vi "TCP通讯.vi"(7 "service name":string caption="服务名称", 8 "error in":errorcluster caption="错误输入（无错误）", 9 "数据输入":string, 10 "选项":enum16{"NA", "侦听", "读取", "写入", "关闭", "打开TCP连接"}(ring)=enum."侦听", 11 "connection ID in":refnum<k5>) -> (0 "error out":errorcluster caption="错误输出", 1 "数据输出":string, 2 "send ok":bool, 3 "connection ID out":refnum<k5>, 4 "open com":bool)   [LabVIEW 2017]
panel:
  out "写入的字节":i32
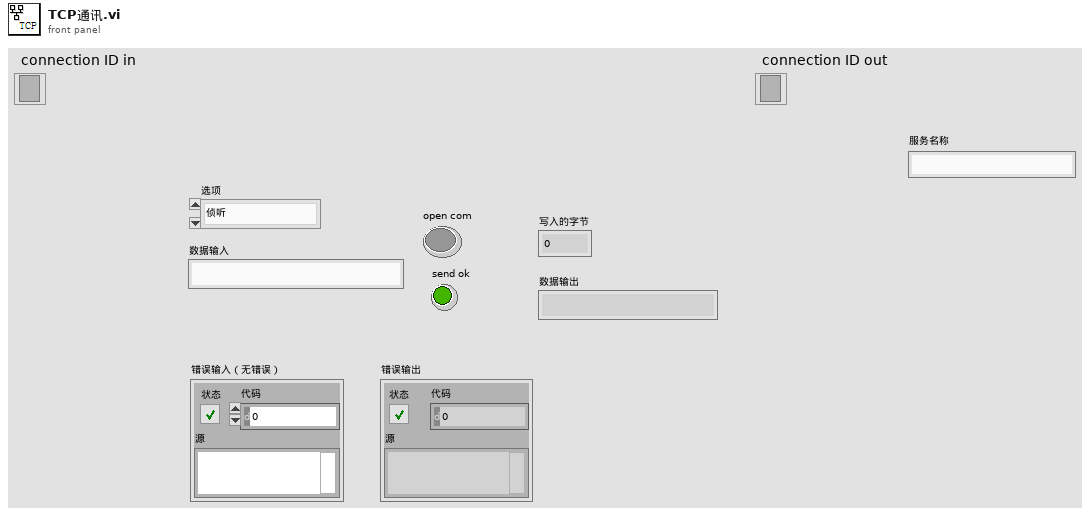
[diagram p1: front panel]
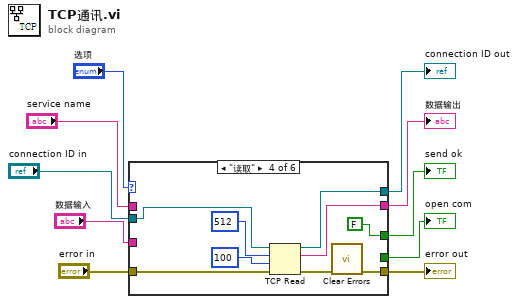
[diagram p0: block diagram]
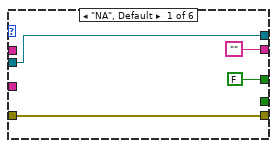
[diagram p2: hidden frame]
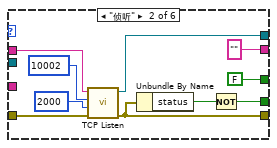
[diagram p3: hidden frame]
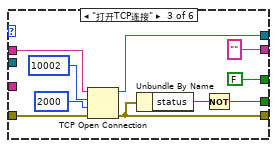
[diagram p4: hidden frame]
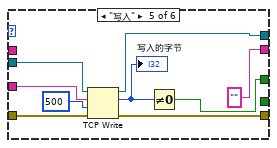
[diagram p5: hidden frame]
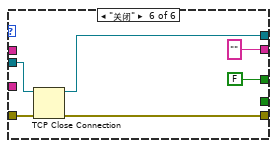
[diagram p6: hidden frame]
diagram:
  n1 = case shown="\"读取\"" "选项" {
    tunnel: [w14 w22 w30 w40 w50 w57] -> w3
    tunnel: "connection ID in" -> [w14 _ _ w41 w51 w58]
    tunnel: "error in" -> [w12 w19 w27 w39 w49 w56]
    tunnel: [w12 w18 w26 w36 w44 w55] -> w8
    tunnel: ["" "" "" w35 "" ""] -> w5
    tunnel: "数据输入" -> [_ _ _ _ w45 _]
    tunnel: [FALSE FALSE FALSE FALSE w48 FALSE] -> w6
    tunnel: [_ w17 w31 _ _ _] -> w4
    tunnel: "service name" -> [_ w15 w25 _ _ _]
    frame "NA", Default {
    }
    frame "侦听" {
      n2 = call <vilib>:"TCP Listen.vi"("error in (no error)"=w19, "timeout ms (wait forever: -1)"=2000, "port"=u16 10002, "service name"=w15) -> ("error out"=w18:errorcluster, "connection ID"=w22:refnum<k5>)  [unwired: 3 in, 3 out]
      n3 = Unbundle By Name(w18) -> ("status"=w23:bool)
      n4 = Not(x=w23) -> (.not. x?=w17:bool)
    }
    frame "打开TCP连接" {
      n5 = TCP Open Connection(address=w25, remote port or service name=u16 10002 ("port"), timeout ms (60000)=2000 ("timeout ms (wait forever: -1)"), error in (no error)=w27) -> (connection ID=w30:refnum<k5>, error out=w26:errorcluster)  [unwired: 1 in]
      n6 = Unbundle By Name(w26) -> ("status"=w34:bool)
      n7 = Not(x=w34) -> (.not. x?=w31:bool)
    }
    frame "读取" {
      n8 = TCP Read(connection ID=w41, bytes to read=512 ("读取的字节"), error in (no error)=w39, 9:100 ("超时毫秒(25000)")) -> (connection ID out=w40:refnum<k5>, data out=w35:string, error out=w37:errorcluster)  [unwired: 1 in]
      n9 = call <vilib>:"Clear Errors.vi"("error in (no error)"=w37) -> ("error out"=w36:errorcluster)  [unwired: 5 in, 1 out]
    }
    frame "写入" {
      n10 = TCP Write(connection ID=w51, data in=w45, error in (no error)=w49, 9:500 ("超时毫秒(25000)")) -> (connection ID out=w50:refnum<k5>, bytes written=w46:i32, error out=w44:errorcluster)
      "写入的字节" <- w46
      n11 = Not Equal To 0?(x=w46) -> (x != 0?=w48:bool)
    }
    frame "关闭" {
      n12 = TCP Close Connection(connection ID=w58, error in (no error)=w56) -> (connection ID out=w57:refnum<k5>, error out=w55:errorcluster)  [unwired: 1 in]
    }
  }
  "数据输出" <- w5
  "error out" <- w8
  "send ok" <- w6
  "open com" <- w4
  "connection ID out" <- w3
